vi "Stop.vi"(8 "error in (no error)":errorcluster, 11 "TimeStamper in":refnum<class "TimeStamper.lvclass">) -> (0 "error out":errorcluster, 3 "TimeStamper out":refnum<class "TimeStamper.lvclass">)   [LabVIEW 2014, in "TimeStamper.lvclass"]
uses:
  TimeStamper.lvclass
  TimeStamper.lvclass/TimeStamper.ctl
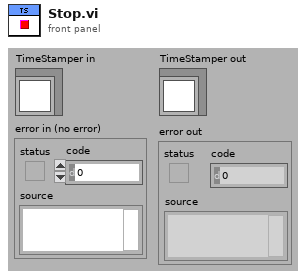
[diagram p1: front panel]
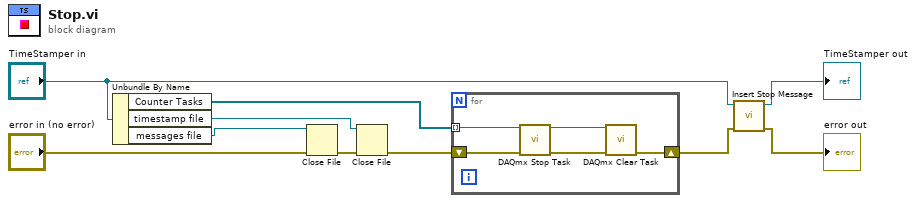
[diagram p0: block diagram]
diagram:
  n1 = Unbundle By Name("TimeStamper in") -> ("Counter Tasks"=w9:refnum<k21>[], "timestamp file"=w8:refnum<file>, "messages file"=w7:refnum<file>)
  n2 = Close File(refnum=w7, error in="error in (no error)") -> (error out=w6:errorcluster)  [unwired: 1 out]
  n3 = Close File(refnum=w8, error in=w6) -> (error out=w5:errorcluster)  [unwired: 1 out]
  n4 = for {
    tunnel: w9 -> [w15] mode=indexing
    shift-right: [w11] -> w3
    shift-left: w5 -> [w12]
    n5 = call <vilib>:"DAQmx Stop Task.vi"("task/channels in"=w15, "error in"=w12) -> ("task out"=w14:refnum<k21>, "error out"=w13:errorcluster)  [unwired: 12 in]
    n6 = call <vilib>:"DAQmx Clear Task.vi"("task in"=w14, "error in"=w13) -> ("error out"=w11:errorcluster)  [unwired: 13 in]
  }
  n7 = call-dynamic "Insert Stop Message.vi"("error in (no error)"=w3, "TimeStamper in"="TimeStamper in") -> ("error out"=→"error out":errorcluster, "TimeStamper out"=→"TimeStamper out":refnum<class "TimeStamper.lvclass">)  [unwired: 8 in]
